vi "U32 to hWnd.vi"(4 "hWnd":u32) -> (1 "hWnd":T1)   [LabVIEW 2011]
uses:
  hWnd.ctl
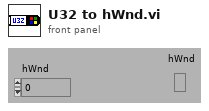
[diagram p1: front panel]
types:
  T1 = typedef "hWnd.ctl" = refnum<k1>
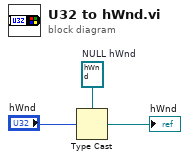
[diagram p0: block diagram]
diagram:
  w1 = T1 refnum  # NULL hWnd
  n1 = Type Cast(type=w1, x="hWnd") -> (*(type *) &x=→"hWnd":T1)
